vi "AlazarEngine.vi"(3 "Imag window array":sgl[](array[numeric]), 4 "Acq Settings":T1={"Window Type"=1, "Record Length"=1536, "Footer"=0, "Output Format"=11, "Offset"=0, "Records Per Buffer"=1000, "Samples per record"=2048, "Records Count (Records/Acq)"=2147483647} {"Window Type" items=["DSP_WINDOW_NONE", "DSP_WINDOW_HANNING", "DSP_WINDOW_HAMMING", "DSP_WINDOW_BLACKMAN", "DSP_WINDOW_BLACKMAN_HARRIS", "DSP_WINDOW_BARTLETT"]; "Footer" items=["FOOTER_NONE", "FOOTER_NPT"]; "Output Format" items=["FLOAT_AMP2"=10, "FLOAT_LOG"=11]}, 5 "Channel":u32(ring)=1 items=["A"=1, "B"=2, "A + B"=3, "C"=4, "A + C"=5, "A + B"=6, "D"=8, "A + D"=9, "B + D"=10, "C + D"=12, "A + B + C + D"=15], 6 "Trigger Settings":T8={"General Trigger Settings"={"Trigger Operation"=0, "Coupling ID"=2, "Range ID"=0, "Delay"=0, "Timeout Ticks"=0, "Mode"=0, "Parameter"=0}, "Trigger Engine 1"={"Trigger Engine"=0, "Source"=0, "Slope"=1, "Level"=0}, "Trigger Engine 2"={"Trigger Engine"=0, "Source"=0, "Slope"=1, "Level"=0}} {"General Trigger Settings"."Trigger Operation" items=["J", "K", "J OR K", "J AND K", "J XOR K", "J AND NOT K", "NOT J AND K"]; "General Trigger Settings"."Coupling ID" items=["AC"=1, "DC"=2]; "General Trigger Settings"."Range ID" items=["5 V", "1 V", "TTL"]; "Trigger Engine 1"."Trigger Engine" items=["J", "K"]; "Trigger Engine 1"."Source" items=["A", "B", "External", "Disable", "C", "D"]; "Trigger Engine 1"."Slope" items=["Positive"=1, "Negative"=2]; "Trigger Engine 2"."Trigger Engine" items=["J", "K"]; "Trigger Engine 2"."Source" items=["A", "B", "External", "Disable", "C", "D"]; "Trigger Engine 2"."Slope" items=["Positive"=1, "Negative"=2]}, 7 "Action":T2=enum."Config Trig", 8 "error in (no error)":errorcluster, 9 "Ch Input Control":T5={"Channel"=1, "Coupling"=2, "Range"=10, "Impedance"=2} {"Channel" items=["A"=1, "B"=2, "C"=4, "D"=8]; "Coupling" items=["AC"=1, "DC"=2]; "Range" items=["20 mV"=1, "40 mV"=2, "50 mV"=3, "80 mV"=4, "100 mV"=5, "200 mV"=6, "400 mV"=7, "500 mV"=8, "800 mV"=9, "1 V"=10, "1.25 V"=33, "2 V"=11, "4 V"=12, "5 V"=13, "8 V"=14, "10 V"=15, "20 V"=16]; "Impedance" items=["1 MOhm"=1, "50 Ohm"=2, ""=0]}, 10 "Capture Clock":T3={"Sample Rate"=30, "Decimation"=0, "Source"=1, "Edge"=0} {"Edge" items=["Rising", "Falling"]; "Source" items=["Internal"=1, "Fast External"=2, "Medium External"=3, "Slow External"=4, "External AC"=5, "External DC"=6, "External 10MHz"=7]}, 11 "Device ID":T4={"System ID"=1, "Board ID"=1}) -> (0 "error out":errorcluster, 2 "Buffer":sgl[](array[numeric]))   [LabVIEW 2018]
uses:
  Controls/General Trigger Settings.ctl
  Controls/Trigger Engine Controls.ctl
  Controls/Channel Input Controls.ctl
  Controls/Alazar Device ID.ctl
  Controls/Clock Controls.ctl
  Controls/Alazar Engine Actions.ctl
  Controls/Alazar Acquisition Settings.ctl
  Controls/Async Read Parameters.ctl
  General/Controls/Queue Manager Actions.ctl
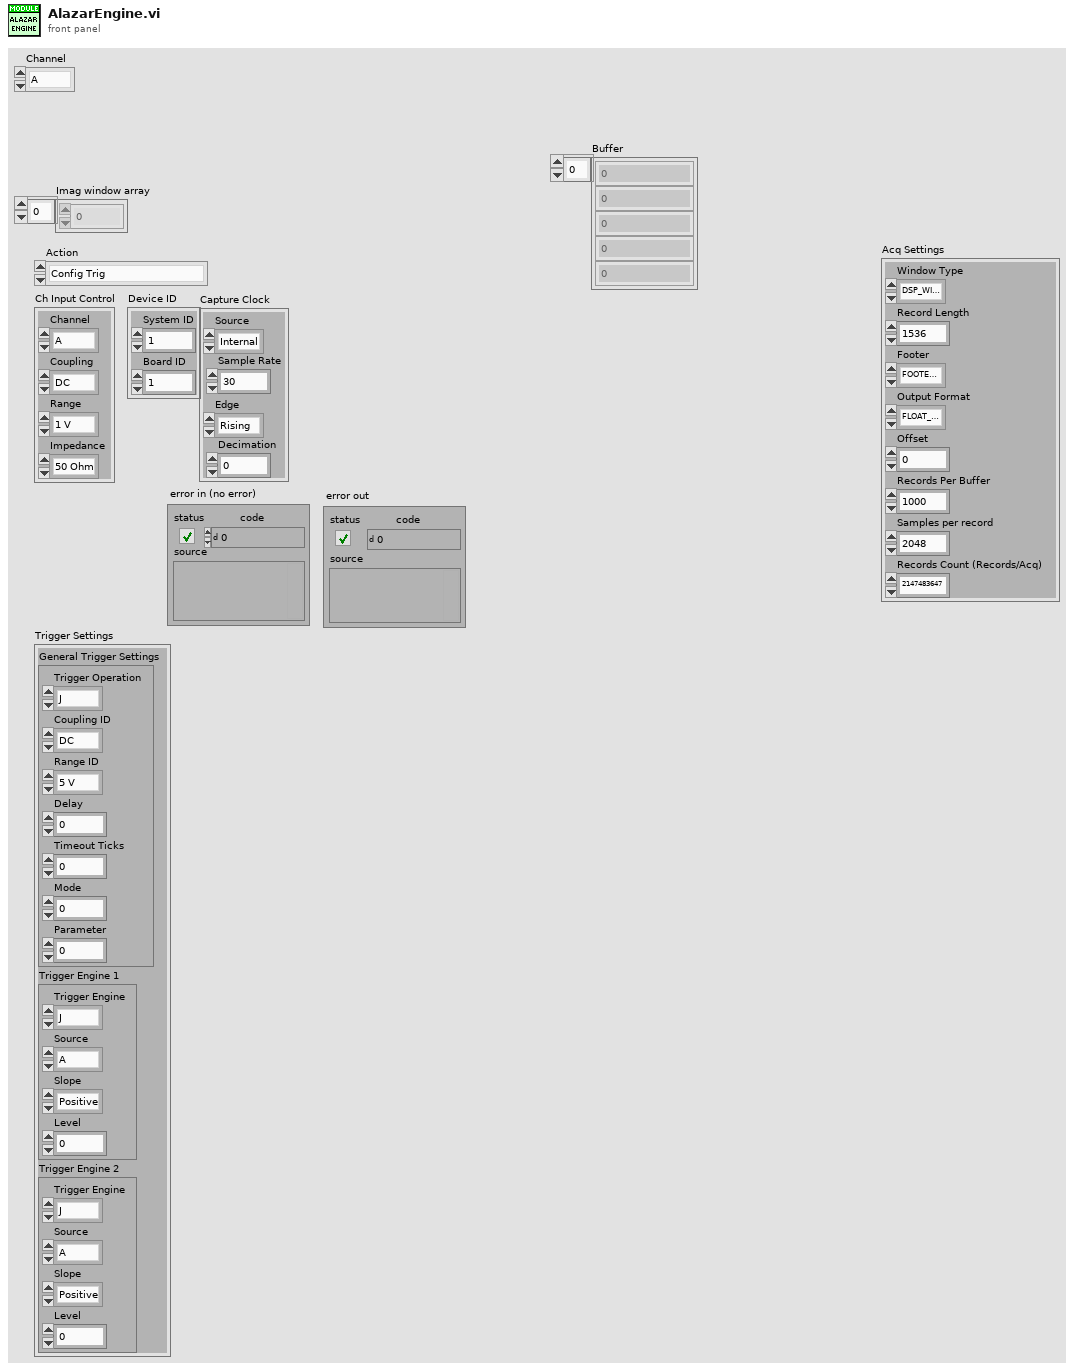
[diagram p1: front panel]
types:
  T1 = typedef "Alazar Acquisition Settings.ctl" = cluster{"Window Type":u32, "Record Length":u32, "Footer":u32, "Output Format":u32, "Offset":u32, "Records Per Buffer":u32, "Samples per record":u32, "Records Count (Records/Acq)":u32}
  T2 = typedef "Alazar Engine Actions.ctl" = enum16{"Init", "Config Clock", "Config Ch", "Config Trig", "Config Non-FFT Acq.", "Non-FFT Acquire", "Load background from Non-FFT buffer", "enable background subtrac", "disable background subtrac", "load background from file", "load background from elsewhere", "start acquire", "background subtraction", "Config Acq.", "Acquire", "UnInit"}
  T3 = typedef "Clock Controls.ctl" = cluster{"Sample Rate":u32, "Decimation":u32, "Source":u32, "Edge":u32}
  T4 = typedef "Alazar Device ID.ctl" = cluster{"System ID":u32, "Board ID":u32}
  T5 = typedef "Channel Input Controls.ctl" = cluster{"Channel":u8, "Coupling":u32, "Range":u32, "Impedance":u32}
  T6 = typedef "General Trigger Settings.ctl" = cluster{"Trigger Operation":u32, "Coupling ID":u32, "Range ID":u32, "Delay":u32, "Timeout Ticks":u32, "Mode":u32, "Parameter":u32}
  T7 = typedef "Trigger Engine Controls.ctl" = cluster{"Trigger Engine":u32, "Source":u32, "Slope":u32, "Level":u32}
  T8 = cluster{"General Trigger Settings":T6, "Trigger Engine 1":T7, "Trigger Engine 2":T7}
  T9 = typedef "Async Read Parameters.ctl" = cluster{"Transfer Offset":u32, "Transfer Length":u32, "Records Per Buffer":u32, "Records Per Acquisition":u32}
  T10 = typedef "Queue Manager Actions.ctl" = enum16{"Init", "Enqueue", "Enqueue All", "Preview Queue", "Dequeue", "Get Status", "Flush Queue", "Flush All Queues", "Release All Queues", "Release Queue", "Enqueue at Opposite End"}
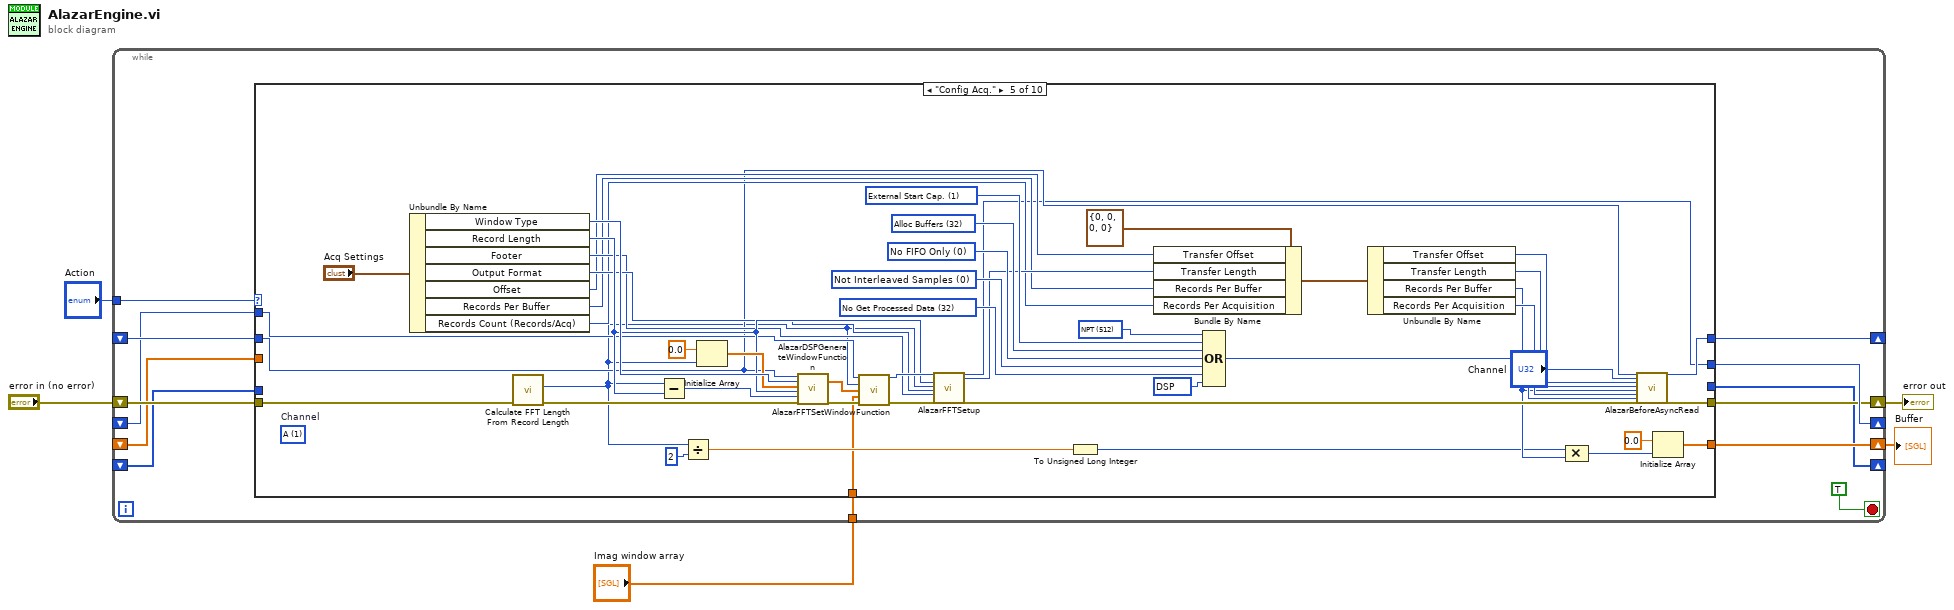
[diagram p0: block diagram]
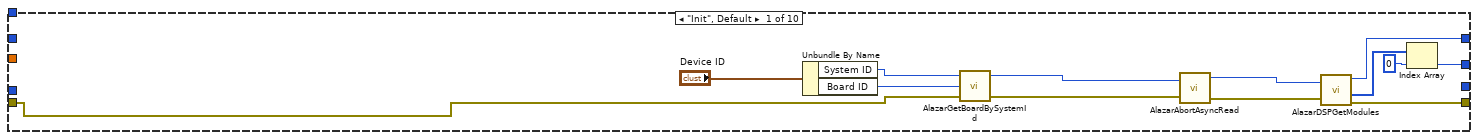
[diagram p2: hidden frame]
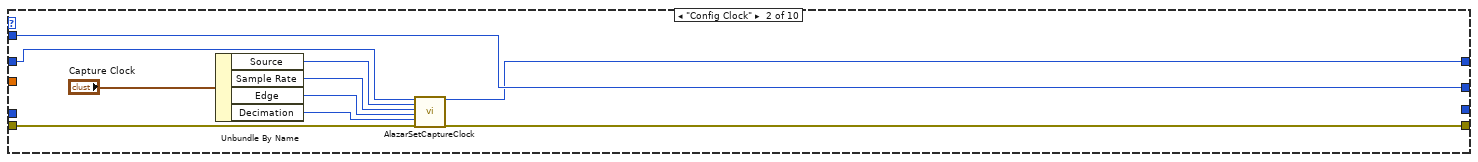
[diagram p3: hidden frame]
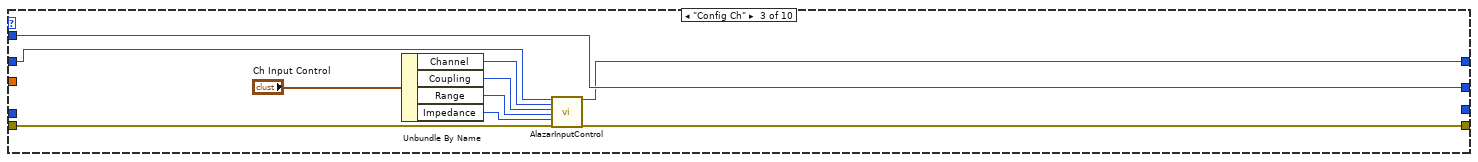
[diagram p4: hidden frame]
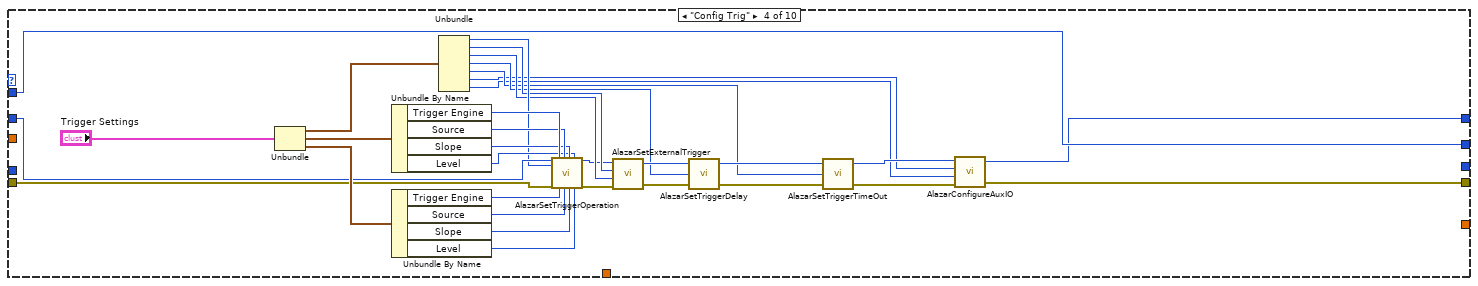
[diagram p5: hidden frame]
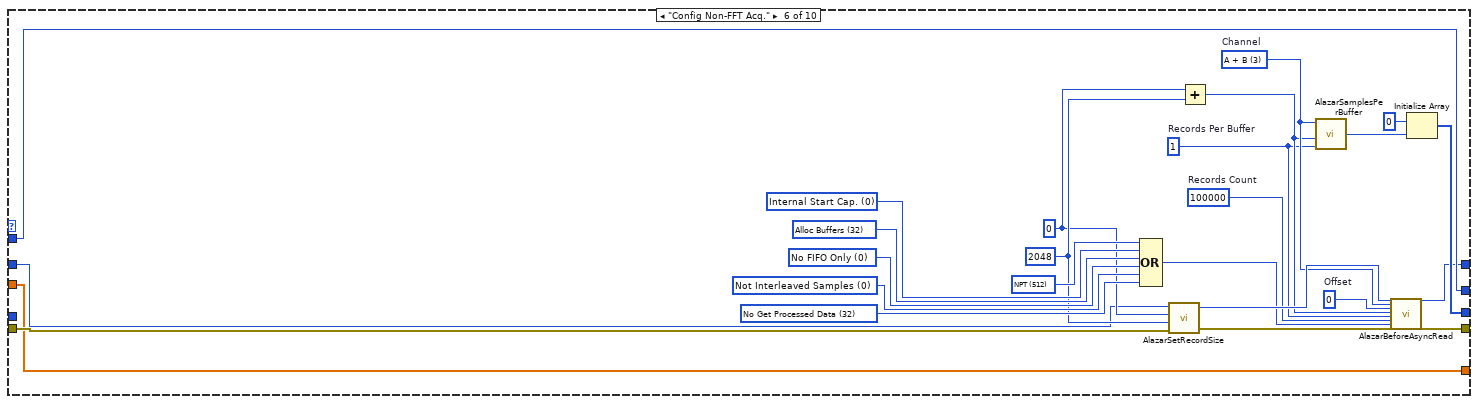
[diagram p6: hidden frame]
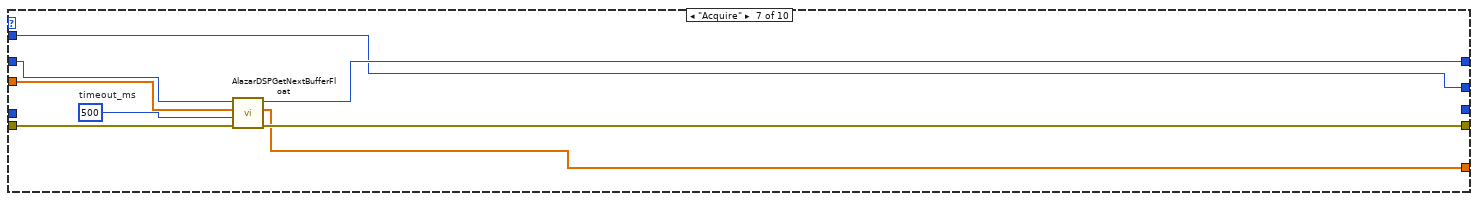
[diagram p7: hidden frame]
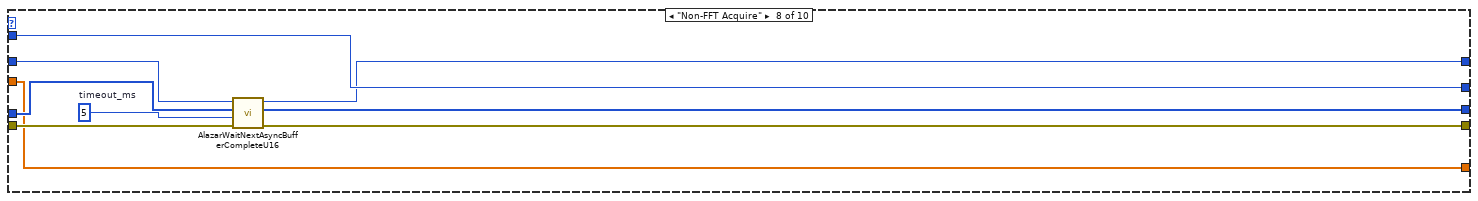
[diagram p8: hidden frame]
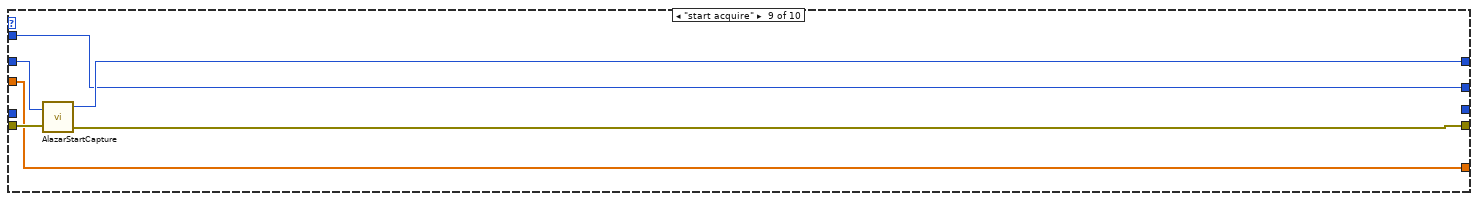
[diagram p9: hidden frame]
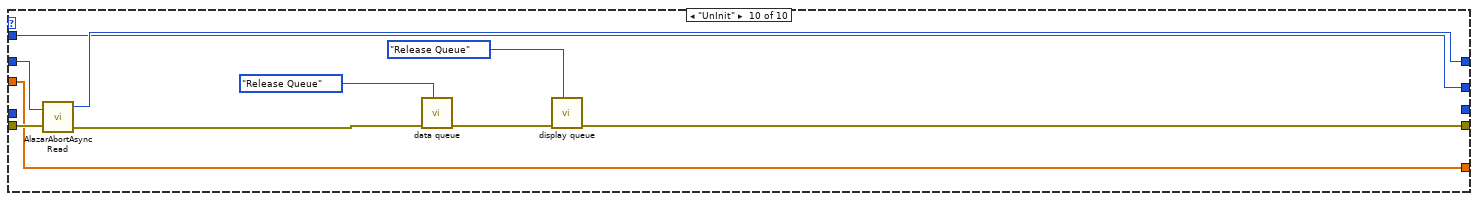
[diagram p10: hidden frame]
diagram:
  n1 = while {
    tunnel: "Action" -> [w16]
    shift-right: [w15] -> _
    shift-left: _ -> [w14]
    shift-right: [w13] -> _
    shift-left: _ -> [w12]
    shift-right: [w11] -> w3
    shift-left: "error in (no error)" -> [w17]
    shift-right: [w10] -> w2
    shift-left: _ -> [w9]
    shift-right: [w8] -> _
    shift-left: _ -> [w7]
    tunnel: "Imag window array" -> [w6]
    stop <- TRUE stop-if-true
    n2 = case shown="\"Config Acq.\"" w16 {
      tunnel: w17 -> [w19 w39 w45 w65 w122 w137 w158 w169 w178 w188]
      tunnel: [w22 w32 w44 w53 w86 w136 w157 w165 w177 w180] -> w11
      tunnel: [w20 w33 w43 w52 w97 w131 w162 w167 w175 w186] -> w15
      tunnel: w14 -> [_ w34 w42 w70 w102 w133 w163 w170 w176 w187]
      tunnel: [w30 w41 w51 w81 w95 w132 w161 w168 w174 w185] -> w13
      tunnel: w12 -> [_ w41 w51 w81 w109 w132 w161 w168 w174 w185]
      tunnel: [_ _ _ _ w88 w134 w156 w166 w173 w184] -> w10
      tunnel: w9 -> [_ _ _ _ _ w134 w159 w166 w173 w184]
      tunnel: [_ _ _ _ _ w135 _ w164 _ _] -> w8
      tunnel: w7 -> [_ _ _ _ _ _ _ w171 _ _]
      tunnel: w6 -> [_ _ _ _ w84 _ _ _ _ _]
      frame "Init", Default {
        n3 = Unbundle By Name("Device ID") -> ("System ID"=w28:u32, "Board ID"=w27:u32)
        n4 = call "AlazarGetBoardBySystemId.vi"("error in (no error)"=w19, "Board ID"=w27, "System ID"=w28) -> ("error out"=w26:errorcluster, "Handle"=w25:u64)  [unwired: 1 out]
        n5 = call "AlazarAbortAsyncRead.vi"("Handle"=w25, "error in (no error)"=w26) -> ("Handle"=w24:u64, "error out"=w23:errorcluster)  [unwired: 1 out]
        n6 = call "AlazarDSPGetModules.vi"("Handle"=w24, "error in (no error)"=w23) -> ("Handle"=w20:u64, "DSP Modules"=w21:u64[], "error out"=w22:errorcluster)  [unwired: 1 out]
        n7 = Index Array(array=w21, index=u32 0) -> (element=w30:u64)
      }
      frame "Config Clock" {
        n8 = Unbundle By Name("Capture Clock") -> ("Source"=w35:u32, "Sample Rate"=w36:u32, "Edge"=w37:u32, "Decimation"=w38:u32)
        n9 = call "AlazarSetCaptureClock.vi"("Handle"=w34, "Source"=w35, "Sample Rate"=w36, "Edge"=w37, "Decimation"=w38, "error in (no error)"=w39) -> ("Handle"=w33:u64, "error out"=w32:errorcluster)  [unwired: 11 in, 1 out]
      }
      frame "Config Ch" {
        n10 = Unbundle By Name("Ch Input Control") -> ("Channel"=w49:u8, "Coupling"=w48:u32, "Range"=w47:u32, "Impedance"=w46:u32)
        n11 = call "AlazarInputControl.vi"("Handle"=w42, "Channel"=w49, "Coupling"=w48, "Range"=w47, "Impedance"=w46, "error in (no error)"=w45) -> ("Handle"=w43:u64, "error out"=w44:errorcluster)  [unwired: 11 in, 1 out]
      }
      frame "Config Trig" {
        n12 = Unbundle("Trigger Settings") -> ("General Trigger Settings"=w82:T6, "Trigger Engine 1"=w80:T7, "Trigger Engine 2"=w79:T7)
        n13 = Unbundle By Name(w80) -> ("Trigger Engine"=w78:u32, "Source"=w77:u32, "Slope"=w76:u32, "Level"=w75:u32)
        n14 = Unbundle By Name(w79) -> ("Trigger Engine"=w74:u32, "Source"=w73:u32, "Slope"=w72:u32, "Level"=w71:u32)
        n15 = Unbundle(w82) -> ("Trigger Operation"=w69:u32, "Coupling ID"=w68:u32, "Range ID"=w67:u32, "Delay"=w61:u32, "Timeout Ticks"=w58:u32, "Mode"=w55:u32, "Parameter"=w54:u32)
        n16 = call "AlazarSetTriggerOperation.vi"("Handle"=w70, "Trigger Operation"=w69, "error in (no error)"=w65, "Trigger Engine 1"=w78, "Trigger Engine 2"=w74, "Source 1"=w77, "Source 2"=w73, "Slope 1"=w76, "Slope 2"=w72, "Level 1"=w75, "Level 2"=w71) -> ("Handle"=w63:u64, "error out"=w66:errorcluster)  [unwired: 6 in, 1 out]
        n17 = call "AlazarSetExternalTrigger.vi"("error in (no error)"=w66, "Range ID"=w67, "Coupling ID"=w68, "Handle"=w63) -> ("error out"=w64:errorcluster, "Handle"=w62:u64)  [unwired: 1 out]
        n18 = call "AlazarSetTriggerDelay.vi"("error in (no error)"=w64, "Delay"=w61, "Handle"=w62) -> ("error out"=w60:errorcluster, "Handle"=w59:u64)  [unwired: 1 out]
        n19 = call "AlazarSetTriggerTimeOut.vi"("error in (no error)"=w60, "Timeout Ticks"=w58, "Handle"=w59) -> ("error out"=w57:errorcluster, "Handle"=w56:u64)  [unwired: 1 out]
        n20 = call "AlazarConfigureAuxIO.vi"("error in (no error)"=w57, "Parameter"=w54, "Mode"=w55, "Handle"=w56) -> ("error out"=w53:errorcluster, "Handle"=w52:u64)  [unwired: 1 out]
      }
      frame "Config Acq." {
        w123 = u32 16384 items=["DSP"=16384]
        (unwired) u32 1 items=["A"=1]  # Channel
        w129 = u32 32 items=["No Get Processed Data"=32, "Get Processed Data"=8192]
        w128 = u32 0 items=["Not Interleaved Samples"=0, "Interleave Samples"=4096]
        w124 = u32 0 items=["No FIFO Only"=0, "FIFO Only"=2048]
        w127 = u32 32 items=["Alloc Buffers"=32]
        w126 = u32 1 items=["Internal Start Cap.", "External Start Cap."]
        w125 = u32 512 items=["Traditional"=0, "NPT"=512, "Continuous"=256, "Triggered Streaming"=1024]
        n21 = Unbundle By Name("Acq Settings") -> ("Window Type"=w119:u32, "Record Length"=w113:u32, "Footer"=w111:u32, "Output Format"=w112:u32, "Offset"=w107:u32, "Records Per Buffer"=w105:u32, "Records Count (Records/Acq)"=w104:u32)
        n22 = call "Calculate FFT Length From Record Length.vi"("error in (no error)"=w122) -> ("error out"=w120:errorcluster, "FFT Length"=w93:u32)  [unwired: 8 in, 1 out]
        n23 = Subtract(x=w93, y=w113) -> (x-y=w118:u32)
        n24 = Divide(x=w93, y=u32 2) -> (x/y=w89:dbl)
        n25 = Initialize Array(sgl 0.0, w93) -> (w116:sgl[])
        n26 = call "AlazarDSPGenerateWindowFunction.vi"("Handle"=w102, "Window Type"=w119, "window"=w116, "WindowLength_samples"=w113, "PaddingLength_samples"=w118, "error in (no error)"=w120) -> ("window"=w117:sgl[], "error out"=w115:errorcluster)  [unwired: 10 in, 2 out]
        n27 = call "AlazarFFTSetWindowFunction.vi"("DSP Handle"=w109, "Samples per record"=w93, "Real window array"=w117, "Imag window array"=w84, "error in (no error)"=w115) -> ("DSP Handle"=w114:u64, "error out"=w110:errorcluster)  [unwired: 9 in]
        n28 = call "AlazarFFTSetup.vi"("DSP Handle"=w114, "Record Length (samples)"=w113, "FFT Length (samples)"=w93, "Output Format"=w112, "Footer"=w111, "error in (no error)"=w110) -> ("DSP Handle"=w95:u64, "Bytes Per Output Record"=w106:u32, "error out"=w96:errorcluster)  [unwired: 18 in, 1 out]
        n29 = To Unsigned Long Integer(number=w89) -> (unsigned 32bit integer=w87:u32)
        n30 = Bundle By Name(cluster=T9 {"Transfer Offset"=0, "Transfer Length"=0, "Records Per Buffer"=0, "Records Per Acquisition"=0} ("ASync Read Parameters"), "Transfer Offset"=w107, "Transfer Length"=w106, "Records Per Buffer"=w105, "Records Per Acquisition"=w104) -> (w103:T9)
        n31 = Compound Arithmetic op=OR(w125, w126, w127, w124, w128, w129, w123) -> (w98:u32)
        n32 = Unbundle By Name(w103) -> ("Transfer Offset"=w101:u32, "Transfer Length"=w100:u32, "Records Per Buffer"=w94:u32, "Records Per Acquisition"=w99:u32)
        n33 = Compound Arithmetic op=MULTIPLY(w87, w94) -> (w92:u32)
        n34 = call "AlazarBeforeAsyncRead.vi"("Handle"=w102, "Channel Select"="Channel", "Transfer Offset"=w101, "Transfer Length"=w100, "Records Per Buffer"=w94, "Records Per Acquisition"=w99, "Flags"=w98, "error in (no error)"=w96) -> ("Handle"=w97:u64, "error out"=w86:errorcluster)  [unwired: 17 in, 1 out]
        n35 = Initialize Array(sgl 0.0 ("element"), w92) -> (w88:sgl[])
      }
      frame "Config Non-FFT Acq." {
        w143 = u32 100000  # Records Count
        w138 = u32 1  # Records Per Buffer
        w144 = u32 0  # Offset
        w140 = u32 3 items=["A"=1, "B"=2, "A + B"=3, "C"=4, "A + C"=5, "A + B"=6, "D"=8, "A + D"=9, "B + D"=10, "C + D"=12, "A + B + C + D"=15]  # Channel
        w149 = u32 2048 ("Post-trigger Samples")
        w148 = u32 0 ("Pre-trigger Samples")
        w155 = u32 32 items=["No Get Processed Data"=32, "Get Processed Data"=8192]
        w154 = u32 0 items=["Not Interleaved Samples"=0, "Interleave Samples"=4096]
        w150 = u32 0 items=["No FIFO Only"=0, "FIFO Only"=2048]
        w153 = u32 32 items=["Alloc Buffers"=32]
        w152 = u32 0 items=["Internal Start Cap.", "External Start Cap."]
        w151 = u32 512 items=["Traditional"=0, "NPT"=512, "Continuous"=256, "Triggered Streaming"=1024]
        n36 = Compound Arithmetic op=OR(w151, w152, w153, w150, w154, w155) -> (w145:u32)
        n37 = call "AlazarSetRecordSize.vi"("error in (no error)"=w137, "Post-trigger Samples"=w149, "Pre-trigger Samples"=w148, "Handle"=w133) -> ("error out"=w146:errorcluster, "Handle"=w147:u64)  [unwired: 1 out]
        n38 = Add(x=w148, y=w149) -> (x+y=w139:u32)
        n39 = call "AlazarSamplesPerBuffer.vi"("Records Per Buffer"=w138, "Samples Per Record"=w139, "Channel Mask"=w140) -> ("Samples Per Buffer"=w141:u32)  [unwired: 1 in]
        n40 = call "AlazarBeforeAsyncRead.vi"("Handle"=w147, "Channel Select"=w140, "Transfer Offset"=w144, "Transfer Length"=w139, "Records Per Buffer"=w138, "Records Per Acquisition"=w143, "Flags"=w145, "error in (no error)"=w146) -> ("Handle"=w131:u64, "error out"=w136:errorcluster)  [unwired: 17 in, 1 out]
        n41 = Initialize Array(u16 0, w141) -> (w135:u16[])
      }
      frame "Acquire" {
        w160 = u32 500  # timeout_ms
        n42 = call "AlazarDSPGetNextBufferFloat.vi"("error in (no error)"=w158, "timeout_ms"=w160, "Buffer"=w159, "Handle"=w163) -> ("error out"=w157:errorcluster, "Buffer"=w156:sgl[], "Handle"=w162:u64)  [unwired: 1 out]
      }
      frame "Non-FFT Acquire" {
        w172 = u32 5  # timeout_ms
        n43 = call "AlazarWaitNextAsyncBufferCompleteU16.vi"("error in (no error)"=w169, "Timeout (ms)"=w172, "Buffer"=w171, "Handle"=w170) -> ("error out"=w165:errorcluster, "Buffer"=w164:u16[], "Handle"=w167:u64)  [unwired: 1 out]
      }
      frame "start acquire" {
        n44 = call "AlazarStartCapture.vi"("Handle"=w176, "error in (no error)"=w178) -> ("Handle"=w175:u64, "error out"=w177:errorcluster)  [unwired: 1 out]
      }
      frame "UnInit" {
        n45 = call "AlazarAbortAsyncRead.vi"("Handle"=w187, "error in (no error)"=w188) -> ("Handle"=w186:u64, "error out"=w183:errorcluster)  [unwired: 1 out]
        n46 = call "data queue.vi"("Action"=Queue_Manager_Actions."Release Queue", "error in (no error)"=w183) -> ("error out"=w181:errorcluster)  [unwired: 6 in, 3 out]
        n47 = call "display queue.vi"("Action"=Queue_Manager_Actions."Release Queue", "error in (no error)"=w181) -> ("error out"=w180:errorcluster)  [unwired: 5 in, 4 out]
      }
    }
  }
  "error out" <- w3
  "Buffer" <- w2
